vi "Build.vi"(8 "error in (no error)":errorcluster, 11 "Project Builder in":refnum<class "Project Builder.lvclass">) -> (0 "error out":errorcluster, 1 "Success?":bool, 3 "Project Builder out":refnum<class "Project Builder.lvclass">)   [LabVIEW 2020, in "ProjectBuilder.lvlib" / "Project Builder.lvclass"]
uses:
  Project Builder.lvclass
  Ctl/Ctl_Build Steps.ctl
  ProjectBuilder.lvlib
  <vilib>/Utility/Data Type/NI_Data Type.lvlib
  PPL/HDH.ClassLoader.lvlibp
  <vilib>/ErrorRing/Error Ring.xnode
  <vilib>/Utility/error.llb/Error Cluster From Error Code.vi
  Project Action/Project Action.lvclass
  Report Action/Report Action/Report Action.lvclass
  C:/Current projects/WS/LV32.2020..ProjectBuilder/Class/Project Action/Project Action.lvclass
panel:
  out "Active Action":string
  out "Sub-Progress":i32(slide) caption="Progress: Sub" scale=0.0..10.0
  out "Progress: Total":i32(slide) scale=0.0..10.0
  out "Active Project":path
  in  "Abort":bool
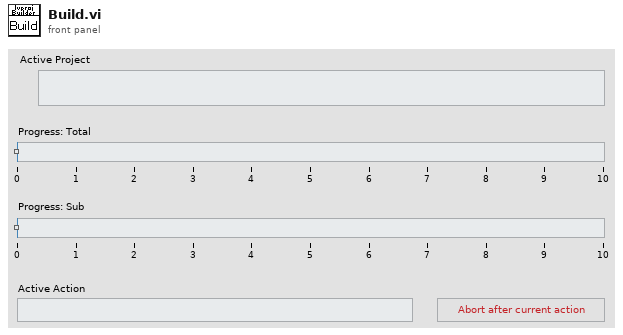
[diagram p1: front panel]
types:
  T1 = typedef "ProjectBuilder.lvlib/Ctl_Build Steps.ctl" = enum16{"Source Test", "Build", "Post-Build Test", "Deploy", "Report"}
  T2 = typedef "ProjectBuilder.lvlib/Project Builder.lvclass/Ctl_Run Cluster.ctl" = cluster{"Source Tests":refnum<class "Project Action.lvclass">[], "Build Array":refnum<class "Project Action.lvclass">[], "Post-Build Tests":refnum<class "Project Action.lvclass">[], "Deploy Array":refnum<class "Project Action.lvclass">[], "Report Handler Array":refnum<class "Report Action.lvclass">[], "Element Count":i32}
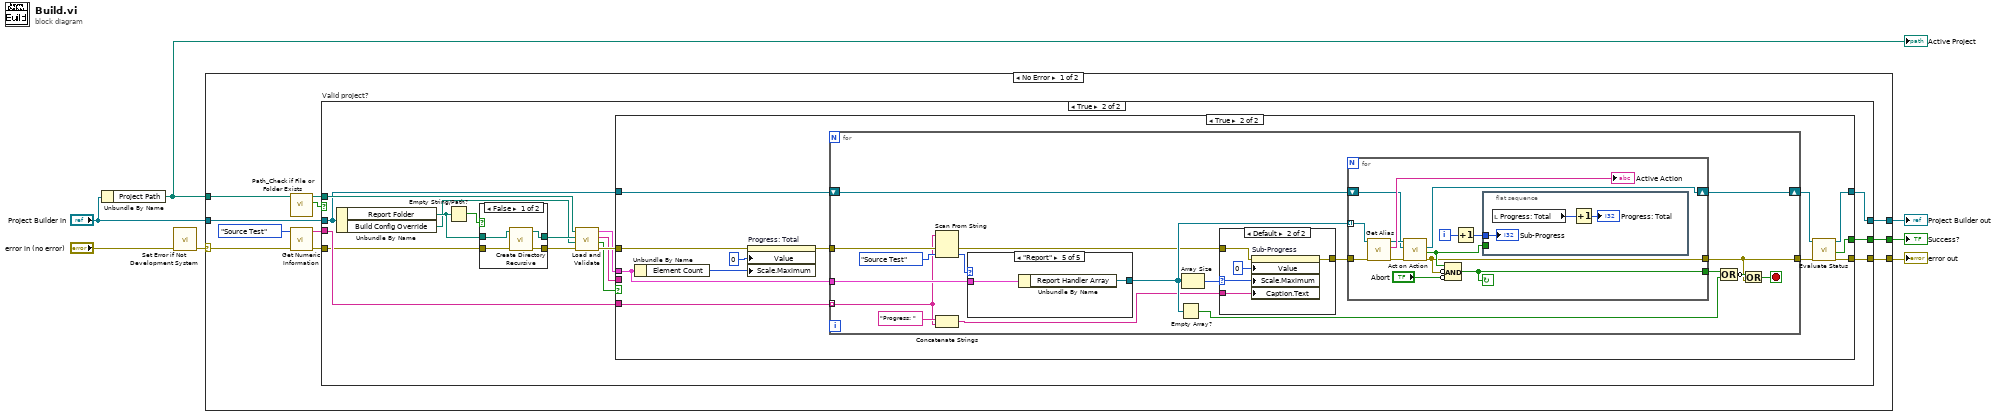
[diagram p0: block diagram]
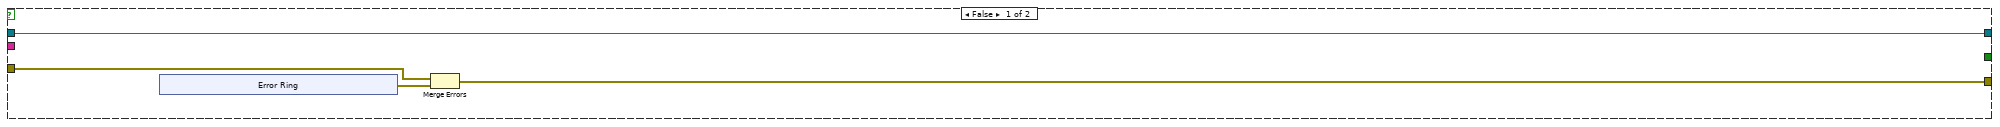
[diagram p2: hidden frame]
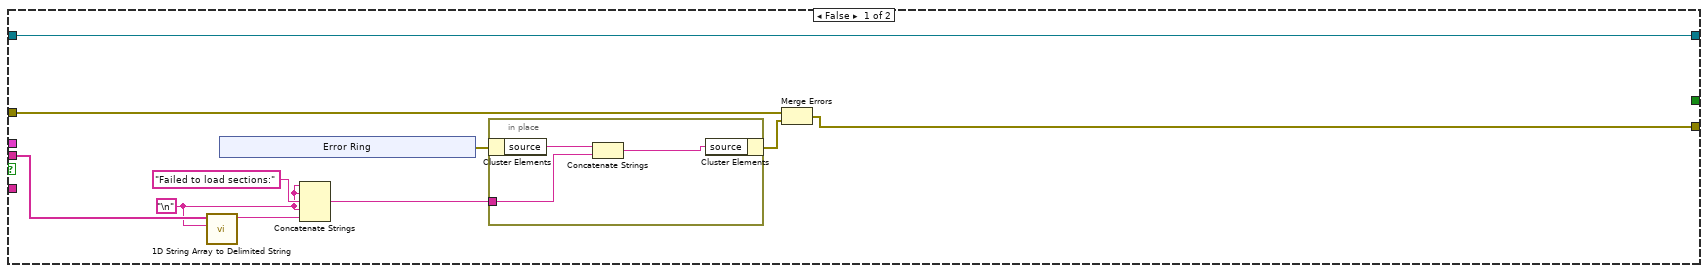
[diagram p4: hidden frame]
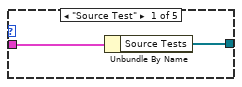
[diagram p6: hidden frame]
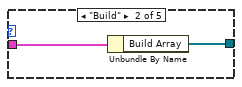
[diagram p7: hidden frame]
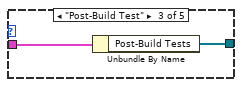
[diagram p8: hidden frame]
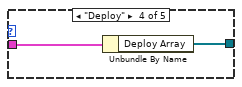
[diagram p9: hidden frame]
diagram:
  n1 = Unbundle By Name("Project Builder in") -> ("Project Path"=w1:path)
  "Active Project" <- w1
  n2 = call "Set Error if Not Development System.vi"("error in (no error)"="error in (no error)") -> ("error out"=w5:errorcluster)  [unwired: 10 in]
  n3 = case shown="No Error" w5 {
    selector: w5 -> [w17 w129]
    tunnel: w1 -> [w18 _]
    tunnel: [w14 w129] -> w7
    tunnel: [w13 _] -> w4
    tunnel: [w8 w128] -> w3
    tunnel: "Project Builder in" -> [w9 w128]
    frame No Error {
      n4 = call "Path_Check if File or Folder Exists.vi"("File or Folder Path in"=w18) -> ("File or Folder Found?"=w16:bool, "File or Folder Path dub"=w15:path)  [unwired: 9 in]
      n5 = call <vilib>:"Get Numeric Information.vi"("error in (no error)"=w17, "variant"=Ctl_Build_Steps."Source Test" ("Build Step")) -> ("error out"=w10:errorcluster, "enum names"=w12:string[])  [unwired: 6 in, 2 out]
      n6 = case "Valid project?" shown="True" w16 {
        tunnel: [w20 w42] -> w14
        tunnel: w10 -> [w22 w30]
        tunnel: w15 -> [_ w41]
        tunnel: [_ w36] -> w13
        tunnel: w12 -> [_ w35]
        tunnel: w9 -> [w19 w33]
        tunnel: [w19 w34] -> w8
        frame False {
          n7 = xnode "Error Ring"() -> ("error out"=w21:errorcluster)
          n8 = Merge Errors(w22, w21) -> (w20:errorcluster)
        }
        frame True {
          n9 = Unbundle By Name(w33) -> ("Report Folder"=w28:path, "Build Config Override"=w27:path)
          n10 = Empty String/Path?(string/path=w28) -> (empty?=w32:bool)
          n11 = case shown="False" w32 {
            tunnel: [w43 w48] -> w31
            tunnel: w30 -> [w46 w48]
            tunnel: [w44 w47] -> w29
            tunnel: w28 -> [w45 w47]
            frame False {
              n12 = call <vilib>:"Create Directory Recursive.vi"("error in (no error)"=w46, "directory"=w45) -> ("error out"=w43:errorcluster, "directory copy"=w44:path)  [unwired: 3 in, 1 out]
            }
            frame True {
            }
          }
          n13 = call "Load and Validate.vi"("error in (no error)"=w31, "Build Config Override"=w27, "Report Folder"=w29, "Project Path"=w41) -> ("error out"=w40:errorcluster, "Valid?"=w38:bool, "Invalid Sections"=w37:string[], "Run cluster"=w39:T2)  [unwired: 4 in]
          n14 = case shown="True" w38 {
            tunnel: [w57 w67] -> w42
            tunnel: w40 -> [w58 w73]
            tunnel: w39 -> [_ w76]
            tunnel: w37 -> [w54 _]
            tunnel: [_ w66] -> w36
            tunnel: w35 -> [_ w77]
            tunnel: [w49 w69] -> w34
            tunnel: w33 -> [w49 w71]
            frame False {
              w50 = "\n"
              n15 = call <vilib>:"1D String Array to Delimited String.vi"("delimiter"=w50, "string array"=w54) -> ("delimited string"=w52:string)  [unwired: 9 in]
              n16 = xnode "Error Ring"() -> ("error out"=w56:errorcluster)
              n17 = Concatenate Strings(w50, w50, "Failed to load sections:", w50, w52) -> (w51:string)
              n18 = in-place {
                in-place-border: w51 -> [w60]
                n19 = in-place-cluster #1(w56) -> ("source"=w61:string)
                n20 = Concatenate Strings(w61, w60) -> (w59:string)
                n21 = in-place-cluster #1("source"=w59) -> (w55:errorcluster)
              }
              n22 = Merge Errors(w58, w55) -> (w57:errorcluster)
            }
            frame True {
              n23 = Unbundle By Name(w76) -> ("Element Count"=w75:i32)
              n24 = property on="Progress: Total" class="Slide (strict)"(error in=w73, "Value"=0 ("Progress: Total"), "Scale.Maximum"=w75) -> (error out=w72:errorcluster)  [unwired: 1 in, 1 out]
              n25 = for {
                tunnel: w72 -> [w88]
                tunnel: [w90] -> w68
                tunnel: w76 -> [w95]
                tunnel: w77 -> [w82] mode=indexing
                shift-right: [w79] -> w70
                shift-left: w71 -> [w80]
                stop <- w92 stop-if-true
                n26 = Scan From String(input string=w82, error in=w88, default 1=Ctl_Build_Steps."Source Test" ("Build Step")) -> (error out=w78:errorcluster, output 1=w87:T1)  [unwired: 2 in, 2 out]
                n27 = Concatenate Strings("Progress: " ("string"), w82) -> (w81:string)
                n28 = case shown="\"Report\"" w87 {
                  tunnel: w95 -> [w119 w121 w123 w125 w127]
                  tunnel: [w118 w120 w122 w124 w126] -> w86
                  frame "Source Test" {
                    n29 = Unbundle By Name(w119) -> ("Source Tests"=w118:refnum<class "Project Action.lvclass">[])
                  }
                  frame "Build" {
                    n30 = Unbundle By Name(w121) -> ("Build Array"=w120:refnum<class "Project Action.lvclass">[])
                  }
                  frame "Post-Build Test" {
                    n31 = Unbundle By Name(w123) -> ("Post-Build Tests"=w122:refnum<class "Project Action.lvclass">[])
                  }
                  frame "Deploy" {
                    n32 = Unbundle By Name(w125) -> ("Deploy Array"=w124:refnum<class "Project Action.lvclass">[])
                  }
                  frame "Report" {
                    n33 = Unbundle By Name(w127) -> ("Report Handler Array"=w126:refnum<class "Report Action.lvclass">[])
                  }
                }
                n34 = Empty Array?(array=w86) -> (empty?=w91:bool)
                n35 = Array Size(array=w86) -> (size(s)=w85:i32)
                n36 = case shown="Default" w85 {
                  selector: w85 -> [_ w100]
                  tunnel: w78 -> [w96 w99]
                  tunnel: [w96 w98] -> w84
                  tunnel: w81 -> [_ w97]
                  frame 0 {
                  }
                  frame Default {
                    n37 = property on="Sub-Progress" class="Slide (strict)"(error in=w99, "Value"=0 ("Progress: Total"), "Scale.Maximum"=w100, "Caption.Text"=w97) -> (error out=w98:errorcluster)  [unwired: 1 in, 1 out]
                  }
                }
                n38 = for {
                  tunnel: w86 -> [w109] mode=indexing
                  tunnel: w84 -> [w114]
                  tunnel: [w102] -> w90
                  tunnel: [w113] -> w94
                  shift-right: [w105] -> w79
                  shift-left: w80 -> [w106]
                  i -> [w111]
                  stop <- w113 continue-if-true
                  n39 = call "Get Alias.vi"("error in (no error)"=w114, "Project Action in"=w109) -> ("error out"=w104:errorcluster, "Alias"=→"Active Action":string, "Project Action out"=w107:refnum<class "Project Action.lvclass">)  [unwired: 7 in]
                  n40 = call "Act on Action.vi"("error in (no error)"=w104, "Project Builder in"=w106, "Project Action in"=w107) -> ("error out"=w102:errorcluster, "Continue?"=w103:bool, "Project Builder out"=w105:refnum<class "Project Builder.lvclass">)  [unwired: 6 in]
                  n41 = Compound Arithmetic op=AND(w103, invert w102, invert "Abort") -> (w113:bool)
                  n42 = Increment(x=w111) -> (x+1=w110:i32)
                  n43 = flat-sequence {
                    tunnel: w110 -> [w117]
                    tunnel: w103 -> [_]
                    frame #0 {
                      n44 = local read "Progress: Total"() -> (w115:i32)
                      n45 = Increment(x=w115) -> (x+1=→"Progress: Total":i32)
                      "Sub-Progress" <- w117
                    }
                  }
                }
                n46 = Compound Arithmetic op=OR(w94, w91) -> (invert w93:bool)
                n47 = Or(x=w93, y=w90) -> (x .or. y?=w92:bool)
              }
              n48 = call "Evaluate Status.vi"("error in (no error)"=w68, "Project Builder in"=w70) -> ("error out"=w67:errorcluster, "Passed?"=w66:bool, "Project Builder out"=w69:refnum<class "Project Builder.lvclass">)  [unwired: 7 in]
            }
          }
        }
      }
    }
    frame Error {
    }
  }
  "error out" <- w7
  "Success?" <- w4
  "Project Builder out" <- w3
